vi "Main.vi"(11 "Module Admin":refnum<class "Delacor_lib_QMH_Module Admin.lvclass">) -> ()   [LabVIEW 2023, in "horiba.lvlib" / "LiveLogger.lvlib"]
doc: "This template is based off of the Queued Message Handler design pattern and the Queued Message Handler project template that ships with LabVIEW.\n\nThe main difference is that the queue is private to this module and communication between modules is performed via Broadcast and Request events.\n\nRequest events are wrapped in public API methods and are handled in the Event Handling Loop (EHL) of this VI. Any module can register for Broadcast events sent by this module. The EHL generates messages based on user interface actions.\n\nThe Message Handling Loop (MHL) processes messages generated by the EHL, or by other messages. The messages are string values, so new messages can be added easily to the Message Cases case structure in the MHL. Each message cluster can also provide an optional value for Message Data, which is a variant that can be converted to whatever message-specific data is required.\n_____\nBased on DQMH Project Template 7.0.1.1316."
uses:
  LiveLogger.lvlib
  <vilib>/Delacor/Delacor QMH/Libraries/Module Admin_class/Delacor_lib_QMH_Module Admin.lvclass
  <vilib>/QSI/QControls/QControl Classes/RichTextBox/Bold Button.ctl
  <vilib>/QSI/QControls/QControl Classes/RichTextBox/Italic Button.ctl
  <vilib>/QSI/QControls/QControl Classes/RichTextBox/Underline Button.ctl
  <vilib>/QSI/QControls/QControl Classes/RichTextBox/Strikethrough Button.ctl
  <vilib>/QSI/QControls/QControl Classes/RichTextBox/Justification.ctl
  <vilib>/QSI/QControls/QControl Classes/RichTextBox/Align Left Button.ctl
  <vilib>/QSI/QControls/QControl Classes/RichTextBox/Align Center Button.ctl
  <vilib>/QSI/QControls/QControl Classes/RichTextBox/Align Right Button.ctl
  <vilib>/QSI/QControls/QControl Classes/RichTextBox/Toggle Codes Button.ctl
  <vilib>/Hampel Software Engineering/HSE Logger/LogLevel.ctl
  Module Data--cluster.ctl
  <vilib>/Delacor/Delacor QMH/Libraries/Message Queue_class/Delacor_lib_QMH_Message Queue.lvclass/Delacor_lib_QMH_Message Queue.ctl
  Stop Argument--cluster.ctl
  <vilib>/Delacor/Delacor QMH/Libraries/Module Admin_class/Delacor_lib_QMH_Module Admin.lvclass/Delacor_lib_QMH_Module Admin.ctl
  <vilib>/Utility/miscctls.llb/LVPointTypeDef.ctl
  <vilib>/Delacor/Delacor QMH/Libraries/Message Queue_class/Delacor_lib_QMH_Enqueue Message (Single).vi
  <vilib>/Delacor/Delacor QMH/Libraries/Module Admin_class/Delacor_lib_QMH_Get External Launch.vi
  <vilib>/Hampel Software Engineering/HSE Logger/Handler/UserEventHandler/UserEventHandler.lvclass
  <vilib>/QSI/QControls/QControl Classes/RichTextBox/RichTextBox.lvclass
  <vilib>/QSI/QControls/QControl Classes/RichTextBox/Write Tagged String.vi
  <vilib>/Delacor/Delacor QMH/Libraries/Message Queue_class/Delacor_lib_QMH_Message Queue.lvclass
  <vilib>/Hampel Software Engineering/HSE Logger/hse-logger.lvlib
panel:
  in  "Autoscroll?":bool
  in  "Toolbar":T7
  in  "RichTextBox":string
  in  "Stop":bool
  out "error out":errorcluster
  in  "Simulate MHL Error":bool
  in  "Simulate EHL Error":bool
  # "Connector Pane"
  # "Locals"
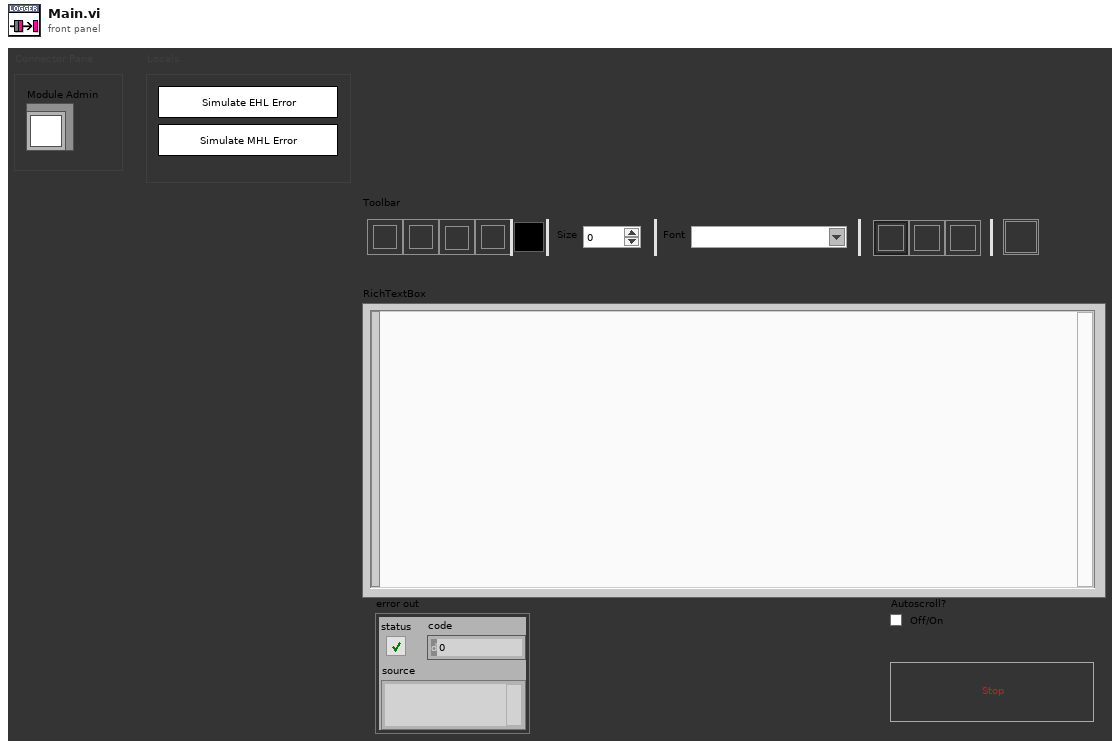
[diagram p1: front panel]
types:
  T1 = typedef "RichTextBox.lvclass/Bold Button.ctl" = bool
  T2 = typedef "RichTextBox.lvclass/Italic Button.ctl" = bool
  T3 = typedef "RichTextBox.lvclass/Underline Button.ctl" = bool
  T4 = typedef "RichTextBox.lvclass/Strikethrough Button.ctl" = bool
  T5 = typedef "RichTextBox.lvclass/Justification.ctl" = enum32{"Left", "Center", "Right"}
  T6 = typedef "RichTextBox.lvclass/Toggle Codes Button.ctl" = bool
  T7 = cluster{"Bold Button":T1, "Italic Button":T2, "Underline Button":T3, "Strikeout Button":T4, "Text Color":u32, "Size":u32, "Font":string, "Justification":T5, "Toggle Codes":T6}
  T8 = typedef "hse-logger.lvlib/LogLevel.ctl" = enum16{"DEBUG", "INFO", "WARNING", "ERROR", "CRITICAL"}
  T9 = typedef "horiba.lvlib/LiveLogger.lvlib/Request Events--cluster.ctl" = cluster{"Stop Module":refnum<user-event>, "Show Panel":refnum<user-event>, "Hide Panel":refnum<user-event>, "Get Module Execution Status":refnum<user-event>, "Show Diagram":refnum<user-event>}
  T10 = typedef "horiba.lvlib/LiveLogger.lvlib/Module Data--cluster.ctl" = cluster{"Status":string}
  T11 = enum32{"invalid lock state", "Not Locked", "Locked (No Password)", "Password-protected"}
  T12 = typedef "horiba.lvlib/LiveLogger.lvlib/Stop Argument--cluster.ctl" = cluster{"Origin":string, "Exit via Stop Module Req?":bool, "Wait for Module to stop?":bool}
  T13 = typedef "LVPointTypeDef.ctl" = cluster{"Horizontal":i16, "Vertical":i16}
  T14 = enum32{"Invalid", "Standard", "Closed", "Hidden", "Minimized", "Maximized"}
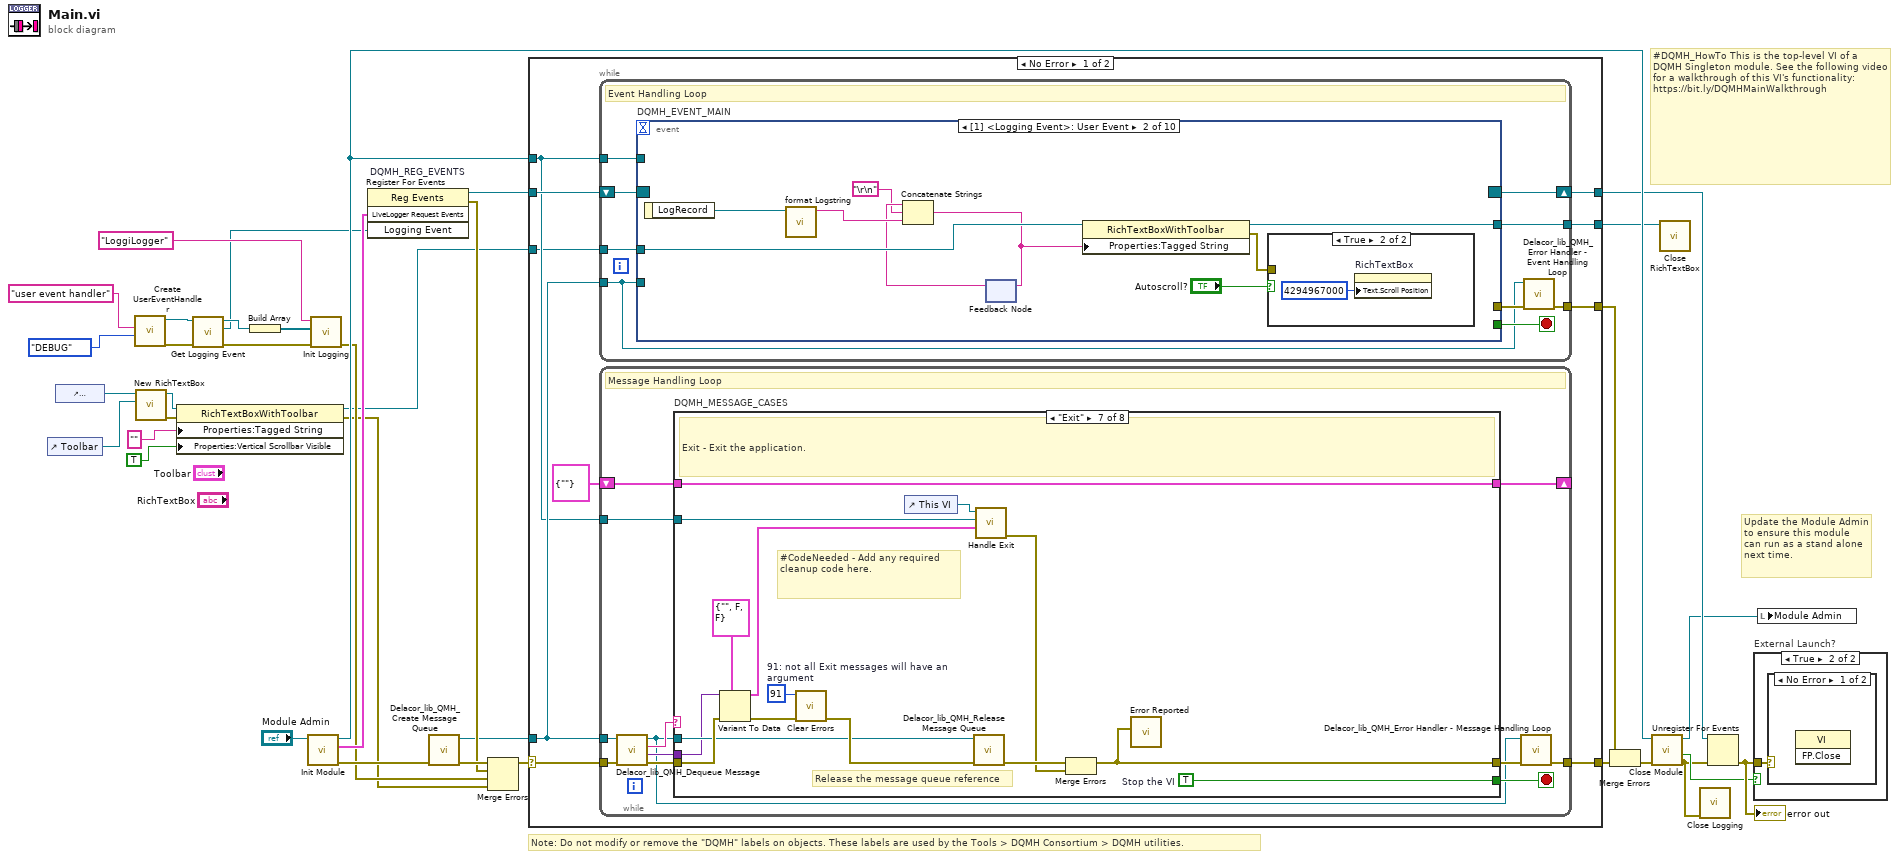
[diagram p0: block diagram]
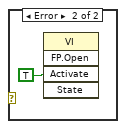
[diagram p3: hidden frame]
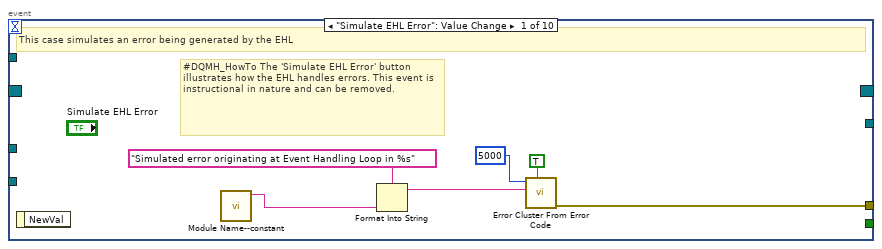
[diagram p4: hidden frame]
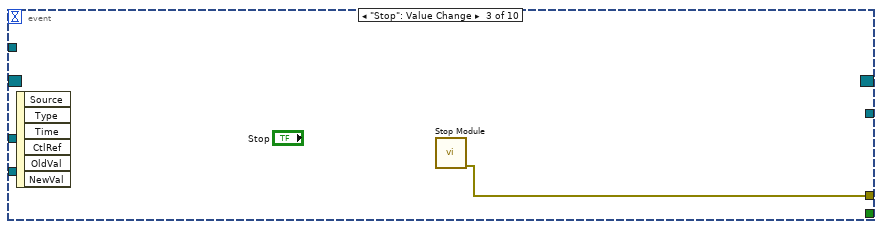
[diagram p6: hidden frame]
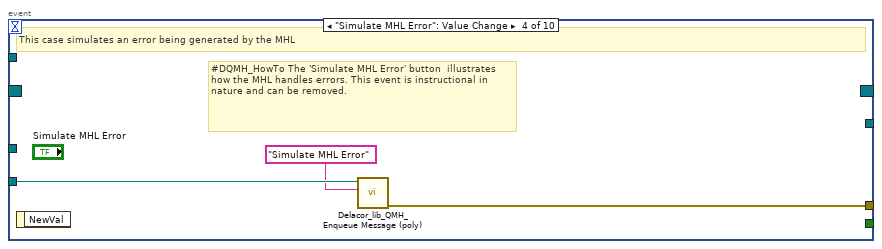
[diagram p7: hidden frame]
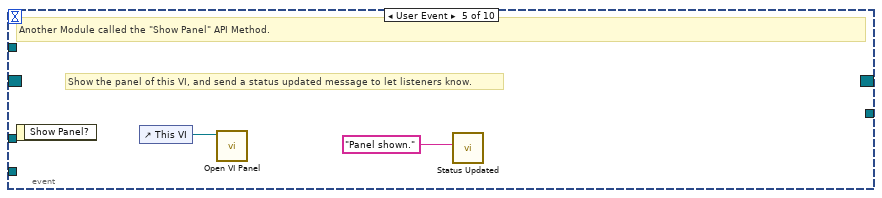
[diagram p8: hidden frame]
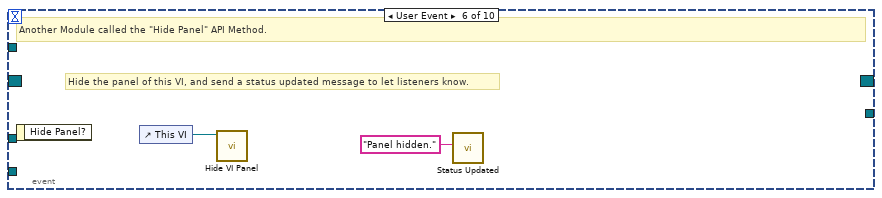
[diagram p9: hidden frame]
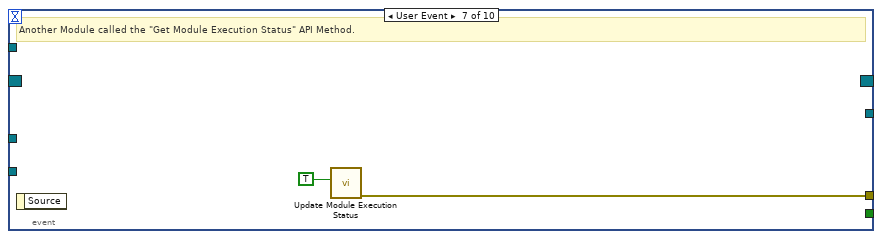
[diagram p10: hidden frame]
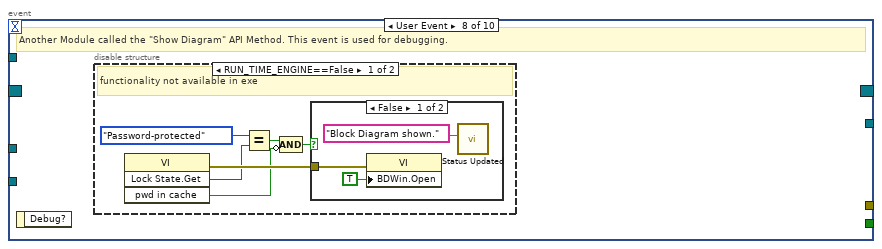
[diagram p11: hidden frame]
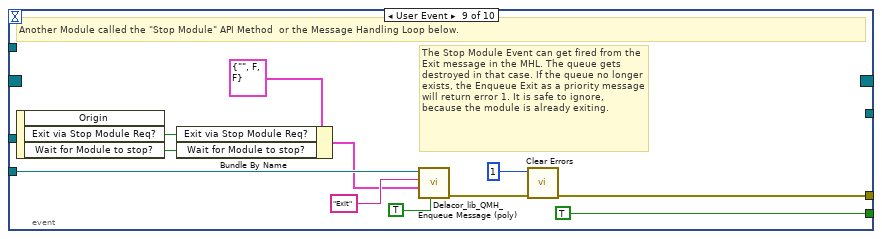
[diagram p14: hidden frame]
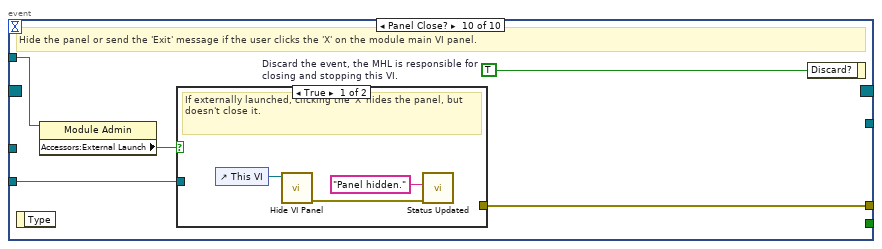
[diagram p15: hidden frame]
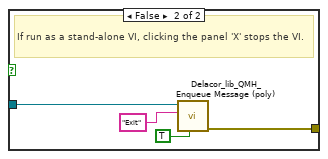
[diagram p16: hidden frame]
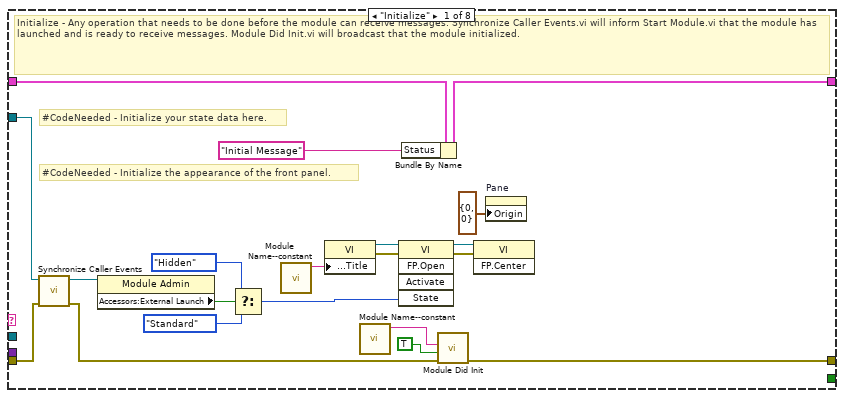
[diagram p17: hidden frame]
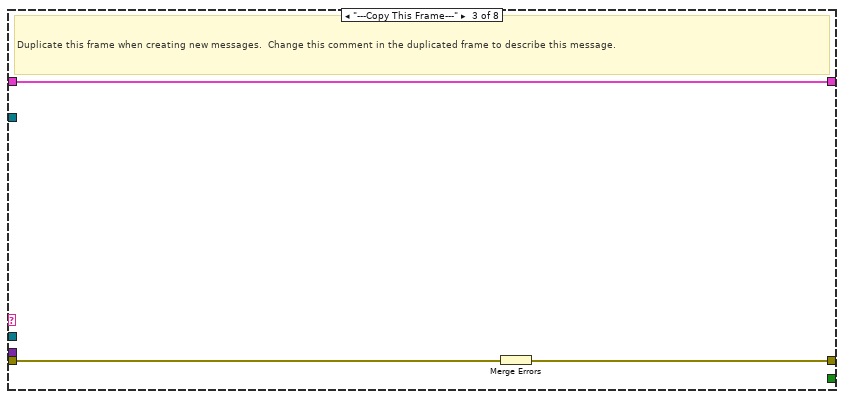
[diagram p19: hidden frame]
diagram:
  # "#DQMH_HowTo This is the top-level VI of a DQMH Singleton module. See the following video for a walkthrough of this VI's functionality: https://bit.ly/DQMHMainWalkthrough"
  # "Note: Do not modify or remove the \"DQMH\" labels on objects. These labels are used by the Tools > DQMH Consortium > DQMH utilities."
  # "Update the Module Admin to ensure this module can run as a stand alone next time."
  n1 = control-ref of="Toolbar"() -> (w8:refnum<vi>)
  n2 = control-ref of="RichTextBox"() -> (w9:refnum<vi>)
  n3 = call <vilib>:"Create UserEventHandler.vi"("Level"=LogLevel."DEBUG", "Name"="user event handler") -> ("error out"=w15:errorcluster, "UserEventHandler out"=w16:refnum<class "UserEventHandler.lvclass">)  [unwired: 8 in]
  n4 = call <vilib>:"New RichTextBox.vi"("ToolbarReference"=w8, "Reference"=w9) -> ("error out"=w7:errorcluster, "RichTextBox out"=w6:refnum<class "RichTextBox.lvclass">)  [unwired: 7 in, 1 out]
  n5 = property class="RichTextBoxWithToolbar"(reference=w6, error in=w7, "Properties:Tagged String"="" ("Status"), "Properties:Vertical Scrollbar Visible"=TRUE ("Vertical Scrollbar Visible")) -> (reference out=w3:refnum<class "RichTextBox.lvclass">, error out=w5:errorcluster)
  n6 = call-dynamic "Get Logging Event.vi"("error in"=w15, "UserEventHandler in"=w16) -> ("error out"=w14:errorcluster, "Logging Event"=w12:refnum<user-event>, "UserEventHandler out"=w13:refnum<class "UserEventHandler.lvclass">)  [unwired: 7 in]
  n7 = Build Array(w13) -> (w19:refnum<class "UserEventHandler.lvclass">[])
  n8 = call "Init Module.vi"("Singleton Module Admin in"="Module Admin") -> ("error out"=w35:errorcluster, "LiveLogger Request Events"=w25:T9, "Singleton Module Admin out"=w28:refnum<class "Delacor_lib_QMH_Module Admin.lvclass">)  [unwired: 8 in]
  n9 = call <vilib>:"Init Logging.vi"("error in"=w14, "Handlers"=w19, "Name"="LoggiLogger") -> ("error out"=w11:errorcluster)  [unwired: 8 in]
  n10 = register-events "DQMH_REG_EVENTS"(w25, w12) -> (reference out=w26:refnum<event-registration>, error out=w29:errorcluster)  [unwired: 2 in]
  n11 = call <vilib>:"Delacor_lib_QMH_Create Message Queue.vi"("error in"=w35) -> ("error out"=w31:errorcluster, "Message Queue"=w24:refnum<class "Delacor_lib_QMH_Message Queue.lvclass">)  [unwired: 9 in]
  n12 = Merge Errors(w31, w29, w11, w5) -> (w30:errorcluster)
  n13 = case shown="No Error" w30 {
    selector: w30 -> [w44 w212]
    tunnel: [w46 w211] -> w36
    tunnel: [w43 w210] -> w27
    tunnel: w26 -> [w41 w210]
    tunnel: w24 -> [w40 w205]
    tunnel: [w45 _] -> w34
    tunnel: w28 -> [w39 w206]
    tunnel: w3 -> [w38 w204]
    tunnel: [w37 w204] -> w2
    frame No Error {
      n14 = while {
        tunnel: w40 -> [w49]
        shift-right: [w52] -> w43
        shift-left: w41 -> [w53]
        tunnel: [w54] -> w45
        tunnel: w39 -> [w50]
        tunnel: w38 -> [w48]
        tunnel: [w47] -> w37
        stop <- w51 stop-if-true
        # "Event Handling Loop"
        n15 = event "DQMH_EVENT_MAIN" shown="[1] <Logging Event>: User Event" {
          selector: w53 -> [_ _ _ _ _ _ _ _ _ _]
          dyn-events: [_ _ _ _ _ _ _ _ _ _] -> w52
          timeout: _ -> [_ _ _ _ _ _ _ _ _ _]
          tunnel: [_ _ _ _ _ _ _ _ TRUE ("Discard?") _] -> w51
          tunnel: w49 -> [_ _ _ w74 _ _ _ _ w97 w104]
          tunnel: [w61 _ w72 w75 _ _ w81 _ w100 w106] -> w55
          tunnel: w50 -> [_ _ _ _ _ _ _ _ _ w103]
          tunnel: w48 -> [_ w68 _ _ _ _ _ _ _ _]
          tunnel: [_ w64 _ _ _ _ _ _ _ _] -> w47
          event "Simulate EHL Error": Value Change {
            # "#DQMH_HowTo The 'Simulate EHL Error' button  illustrates how the EHL handles errors. This event is instructional in nature and can be removed."
            # "This case simulates an error being generated by the EHL"
            n16 = event-data() -> ()  [unwired: 1 in, 1 out]
            n17 = call "Module Name--constant.vi"() -> ("Module Name"=w58:string)  [unwired: 11 in]
            n18 = Format Into String(format string="Simulated error originating at Event Handling Loop in %s", w58) -> (resulting string=w59:string)  [unwired: 2 in, 1 out]
            n19 = call <vilib>:"Error Cluster From Error Code.vi"("show call chain? (False)"=TRUE, "error message (\"\")"=w59, "error code (0)"=5000) -> ("error out"=w61:errorcluster)  [unwired: 6 in]
          }
          event User Event {
            n20 = event-data() -> ("LogRecord"=w70:refnum<class "LogRecord.lvclass">)  [unwired: 1 in]
            n21 = call "format Logstring.vi"("LogRecord in"=w70) -> ("LogLine"=w69:string)  [unwired: 10 in]
            n22 = feedback #1() -> (w67:string)  [unwired: 1 in]
            n23 = Concatenate Strings(w67, "\r\n", w69) -> (w65:string)
            n24 = feedback-in #1(w65) -> ()
            n25 = property class="RichTextBoxWithToolbar"(reference=w68, "Properties:Tagged String"=w65) -> (reference out=w64:refnum<class "RichTextBox.lvclass">, error out=w62:errorcluster)  [unwired: 1 in]
            n26 = case shown="True" "Autoscroll?" {
              tunnel: w62 -> [_ _]
              frame False {
              }
              frame True {
                n27 = property on="RichTextBox" class="Str"("Text.Scroll Position"=u32 4294967000) -> ()  [unwired: 2 in, 2 out]
              }
            }
          }
          event "Stop": Value Change {
            n28 = event-data() -> ()  [unwired: 1 in, 6 out]
            n29 = call "Stop Module.vi"() -> ("error out"=w72:errorcluster)  [unwired: 11 in]
          }
          event "Simulate MHL Error": Value Change {
            # "#DQMH_HowTo The 'Simulate MHL Error' button  illustrates how the MHL handles errors. This event is instructional in nature and can be removed."
            # "This case simulates an error being generated by the MHL"
            n30 = event-data() -> ()  [unwired: 1 in, 1 out]
            n31 = call-poly <vilib>:"Delacor_lib_QMH_Enqueue Message (poly).vi"("Message"="Simulate MHL Error", "Message Queue in"=w74) -> ("error out"=w75:errorcluster)  [unwired: 8 in, 1 out]
          }
          event User Event {
            # "Show the panel of this VI, and send a status updated message to let listeners know."
            # "Another Module called the \"Show Panel\" API Method."
            n32 = event-data() -> ()  [unwired: 1 in, 1 out]
            n33 = control-ref of="This VI"() -> (w77:refnum<vi>)
            n34 = call "Open VI Panel.vi"("VI"=w77) -> ()  [unwired: 10 in, 1 out]
            n35 = call "Status Updated.vi"("Status"="Panel shown." ("format string")) -> ()  [unwired: 10 in, 1 out]
          }
          event User Event {
            # "Hide the panel of this VI, and send a status updated message to let listeners know."
            # "Another Module called the \"Hide Panel\" API Method."
            n36 = event-data() -> ()  [unwired: 1 in, 1 out]
            n37 = control-ref of="This VI"() -> (w79:refnum<vi>)
            n38 = call "Hide VI Panel.vi"("VI"=w79) -> ()  [unwired: 10 in, 1 out]
            n39 = call "Status Updated.vi"("Status"="Panel hidden." ("format string")) -> ()  [unwired: 10 in, 1 out]
          }
          event User Event {
            # "Another Module called the \"Get Module Execution Status\" API Method."
            n40 = event-data() -> ()  [unwired: 1 in, 1 out]
            n41 = call "Update Module Execution Status.vi"("Running?"=TRUE) -> ("error out"=w81:errorcluster)  [unwired: 10 in]
          }
          event User Event {
            # "Another Module called the \"Show Diagram\" API Method. This event is used for debugging."
            n42 = event-data() -> ()  [unwired: 1 in, 1 out]
            n43 = disable-structure shown="RUN_TIME_ENGINE==False" {
              frame condition #0 (active) {
                # "functionality not available in exe"
                n44 = invoke on="Invoke Node" class="VI" method="Lock State.Get"() -> (error out=w87:errorcluster, "Get Lock State"=w86:T11, "pwd in cache"=w83:bool)  [unwired: 4 in, 1 out]
                n45 = Equal?(x=T11."Password-protected", y=w86) -> (x = y?=w84:bool)
                n46 = Compound Arithmetic op=AND(w84, invert w83) -> (w82:bool)
                n47 = case shown="False" w82 {
                  tunnel: w87 -> [w90 _]
                  frame False {
                    n48 = property on="Property Node" class="VI"(error in=w90, "BDWin.Open"=TRUE ("Block Diagram Window:Open")) -> ()  [unwired: 1 in, 2 out]
                    n49 = call "Status Updated.vi"("Status"="Block Diagram shown." ("format string")) -> ()  [unwired: 10 in, 1 out]
                  }
                  frame True {
                    # "Password-protected VI, and the password is not in the cache. Do not show the diagram."
                  }
                }
              }
              frame condition #1 {
              }
            }
          }
          event User Event {
            # "The Stop Module Event can get fired from the Exit message in the MHL. The queue gets destroyed in that case. If the queue no longer exists, the Enqueue Exit as a priority message will return error 1. It is safe to ignore, because the module is already exiting."
            # "Another Module called the \"Stop Module\" API Method  or the Message Handling Loop below."
            n50 = event-data() -> ("Exit via Stop Module Req?"=w93:bool, "Wait for Module to stop?"=w92:bool)  [unwired: 1 in, 1 out]
            n51 = Bundle By Name(cluster=T12 {"Origin"="", "Exit via Stop Module Req?"=FALSE, "Wait for Module to stop?"=FALSE} ("Stop Argument"), "Exit via Stop Module Req?"=w93, "Wait for Module to stop?"=w92) -> (w91:T12)
            n52 = call-poly <vilib>:"Delacor_lib_QMH_Enqueue Message (poly).vi"("Priority Message? (F)"=TRUE, "Message Data"=w91, "Message"="Exit", "Message Queue in"=w97) -> ("error out"=w101:errorcluster)  [unwired: 6 in, 1 out]
            n53 = call <vilib>:"Clear Errors.vi"("error in (no error)"=w101, "specific error code to clear (0: all)"=1) -> ("error out"=w100:errorcluster)  [unwired: 4 in, 1 out]
          }
          event Panel Close? {
            w105 = TRUE  # Discard the event, the MHL is responsible for closing and stopping this VI.
            # "Hide the panel or send the 'Exit' message if the user clicks the 'X' on the module main VI panel."
            n54 = event-data() -> ()  [unwired: 1 in, 1 out]
            n55 = property on="Property Node" class="Module Admin"(reference=w103) -> ("Accessors:External Launch"=w102:bool)  [unwired: 1 in, 2 out]
            n56 = case shown="True" w102 {
              tunnel: w104 -> [_ w112]
              tunnel: [_ w113] -> w106
              frame True {
                # "If externally launched, clicking the 'X' hides the panel, but doesn't close it."
                n57 = control-ref of="This VI"() -> (w109:refnum<vi>)
                n58 = call "Hide VI Panel.vi"("VI"=w109) -> ("error out"=w107:errorcluster)  [unwired: 10 in]
                n59 = call "Status Updated.vi"("error in"=w107, "Status"="Panel hidden." ("format string")) -> ()  [unwired: 9 in, 1 out]
              }
              frame False {
                # "If run as a stand-alone VI, clicking the panel 'X' stops the VI."
                n60 = call-poly <vilib>:"Delacor_lib_QMH_Enqueue Message (poly).vi"("Priority Message? (F)"=TRUE, "Message"="Exit", "Message Queue in"=w112) -> ("error out"=w113:errorcluster)  [unwired: 7 in, 1 out]
              }
            }
            n61 = event-data ("Event Filter Node")("Discard?"=w105) -> ()  [unwired: 1 in, 1 out]
          }
        }
        n62 = call-dynamic "Delacor_lib_QMH_Error Handler - Event Handling Loop.vi"("error in"=w55, "Message Queue in"=w49) -> ("dup error in"=w54:errorcluster)  [unwired: 8 in, 1 out]
      }
      n63 = while {
        tunnel: w40 -> [w114]
        shift-right: [w122] -> _
        shift-left: T10 {"Status"=""} ("Data Cluster") -> [w123]
        tunnel: w44 -> [w125]
        tunnel: [w117] -> w46
        tunnel: w39 -> [w118]
        stop <- w121 stop-if-true
        # "Message Handling Loop"
        n64 = call-dynamic "Delacor_lib_QMH_Dequeue Message.vi"("error in"=w125, "Message Queue in"=w114) -> ("error out"=w124:errorcluster, "Message Data"=w119:variant, "Message"=w120:string, "Message Queue out"=w115:refnum<class "Delacor_lib_QMH_Message Queue.lvclass">)  [unwired: 6 in]
        n65 = case "DQMH_MESSAGE_CASES" shown="\"Exit\"" w120 {
          selector: w120 -> [_ _ _ _ _ _ _ w199]
          tunnel: w115 -> [_ _ _ _ _ w165 w187 _]
          tunnel: w124 -> [w143 w147 w150 w152 w161 w172 w193 w202]
          tunnel: [w141 w147 w149 w152 w160 w168 w188 w203] -> w116
          tunnel: w123 -> [w132 w146 w148 w151 w158 w167 w186 w200]
          tunnel: [w131 w146 w148 w151 w158 w167 w186 w200] -> w122
          tunnel: [_ _ _ _ _ _ w185 _] -> w121
          tunnel: w119 -> [_ _ _ _ _ w166 w184 _]
          tunnel: w118 -> [w133 _ _ _ _ w164 w179 _]
          frame "Initialize" {
            # "#CodeNeeded - Initialize the appearance of the front panel."
            # "#CodeNeeded - Initialize your state data here."
            # "Initialize - Any operation that needs to be done before the module can receive messages. Synchronize Caller Events.vi will inform Start Module.vi that the module has launched and is ready to receive messages. Module Did Init.vi will broadcast that the module initialized."
            n66 = call "Synchronize Caller Events.vi"("error in"=w143, "Singleton Module Admin in"=w133) -> ("error out"=w142:errorcluster, "Singleton Module Admin out"=w128:refnum<class "Delacor_lib_QMH_Module Admin.lvclass">)  [unwired: 8 in]
            n67 = property on="Property Node" class="Module Admin"(reference=w128) -> ("Accessors:External Launch"=w137:bool)  [unwired: 1 in, 2 out]
            n68 = Select(t=T14."Hidden" ("State"), s=w137, f=T14."Standard" ("State")) -> (s? t:f=w134:T14)
            n69 = call "Module Name--constant.vi"() -> ("Module Name"=w140:string)  [unwired: 11 in]
            n70 = property on="Property Node" class="VI"("Front Panel.Title"=w140) -> (reference out=w139:refnum<vi>, error out=w145:errorcluster)  [unwired: 2 in]
            n71 = call "Module Name--constant.vi"() -> ("Module Name"=w129:string)  [unwired: 11 in]
            n72 = invoke on="Invoke Node" class="VI" method="FP.Open"(reference=w139, error in=w145, "State"=w134) -> (reference out=w138:refnum<vi>, error out=w144:errorcluster)  [unwired: 2 in, 3 out]
            n73 = Bundle By Name(cluster=w132, "Status"="Initial Message" ("Initial Message")) -> (w131:T10)
            n74 = call "Module Did Init.vi"("error in"=w142, "Initialized?"=TRUE, "Origin"=w129) -> ("error out"=w141:errorcluster)  [unwired: 8 in]
            n75 = invoke on="Invoke Node" class="VI" method="FP.Center"(reference=w138, error in=w144) -> ()  [unwired: 1 in, 3 out]
            n76 = property on="Pane" class="Pane"("Origin"=T13 {"Horizontal"=0, "Vertical"=0}) -> ()  [unwired: 2 in, 2 out]
          }
          frame "---Module Specific---" {
            # "Separator -- The following cases handle messages specific to this Module."
          }
          frame "---Copy This Frame---" {
            # "Duplicate this frame when creating new messages.  Change this comment in the duplicated frame to describe this message."
            n77 = Merge Errors(w150) -> (w149:errorcluster)
          }
          frame "---Exit and Error Handling---" {
            # "Separator - The following cases handle errors and exit messages."
          }
          frame "Simulate MHL Error" {
            # "#DQMH_HowTo The 'Simulate MHL Error' button  illustrates how the MHL handles errors. This event is instructional in nature and can be removed."
            # "Simulate an error occurring at the MHL"
            n78 = call "Module Name--constant.vi"() -> ("Module Name"=w154:string)  [unwired: 11 in]
            n79 = Format Into String(format string="Simulated error originating at Message Handling Loop in %s", w154) -> (resulting string=w155:string)  [unwired: 2 in, 1 out]
            n80 = call <vilib>:"Error Cluster From Error Code.vi"("show call chain? (False)"=TRUE, "error message (\"\")"=w155, "error code (0)"=5001) -> ("error out"=w159:errorcluster)  [unwired: 6 in]
            n81 = Merge Errors(w161, w159) -> (w160:errorcluster)
          }
          frame "Error" {
            # "#CodeRecommended - If the module is running in standalone mode (External Launch = FALSE), this code will pop up an error dialog and call the 'Exit' message if an error occurs. Add more fine-grained error management here."
            # "Error - Check the error message data and respond accordingly. This message is sent by the \"Error Handler\" VIs at the end of each loop in this application."
            n82 = property on="Property Node" class="Module Admin"(reference=w164) -> ("Accessors:External Launch"=w163:bool)  [unwired: 1 in, 2 out]
            n83 = Variant To Data(error in=w172, type=errorcluster {"status"=FALSE, "code"=0, "source"=""} ("error constant"), Variant=w166) -> (data=w162:errorcluster, error out=w170:errorcluster)
            n84 = local write "error out"(w162) -> ()
            n85 = call "Error Reported.vi"("Error"=w162) -> ()  [unwired: 10 in, 1 out]
            n86 = case shown="False" w163 {
              tunnel: [w177 _] -> w169
              tunnel: w165 -> [w175 _]
              tunnel: w162 -> [w176 _]
              frame False {
                n87 = disable-structure shown="Default" {
                  disable-tunnel: w176 -> [w178 _]
                  frame condition #0 (active) {
                    # "If the module is running standalone, then pop up an error dialog and call the \"Exit\" message."
                    n88 = call <vilib>:"Simple Error Handler.vi"("error in (no error)"=w178) -> ()  [unwired: 4 in, 5 out]
                  }
                  frame condition #1 {
                    # "To prevent the Simple Error Handler VI from being loaded (e.g. when deploying to a Real-Time target), add the Conditional Disable Symbol \"DQMH_Disable_SEH\" to your project and set it to TRUE."
                  }
                }
                n89 = call-poly <vilib>:"Delacor_lib_QMH_Enqueue Message (poly).vi"("Priority Message? (F)"=TRUE, "Message"="Exit", "Message Queue in"=w175) -> ("error out"=w177:errorcluster)  [unwired: 7 in, 1 out]
              }
              frame True {
                # "If the module was launched externally, calling the Error Reported broadcast VI is the only action performed by the \"Error\" message. The module's caller can then process the error appropriately."
              }
            }
            n90 = Merge Errors(w170, w169) -> (w168:errorcluster)
          }
          frame "Exit" {
            w183 = 91  # 91: not all Exit messages will have an argument
            w185 = TRUE  # Stop the VI
            # "Release the message queue reference"
            # "#CodeNeeded - Add any required cleanup code here."
            # "Exit - Exit the application."
            n91 = Variant To Data(error in=w193, type=T12 {"Origin"="", "Exit via Stop Module Req?"=FALSE, "Wait for Module to stop?"=FALSE} ("Stop Argument"), Variant=w184) -> (data=w181:T12, error out=w190:errorcluster)
            n92 = call <vilib>:"Clear Errors.vi"("error in (no error)"=w190, "specific error code to clear (0: all)"=w183) -> ("error out"=w192:errorcluster)  [unwired: 4 in, 1 out]
            n93 = control-ref of="This VI"() -> (w180:refnum<vi>)
            n94 = call-dynamic "Delacor_lib_QMH_Release Message Queue.vi"("error in"=w192, "Message Queue"=w187) -> ("error out"=w191:errorcluster)  [unwired: 9 in]
            n95 = call "Handle Exit.vi"("Stop Argument"=w181, "Admin in"=w179, "VI reference"=w180) -> ("error out"=w189:errorcluster)  [unwired: 7 in, 1 out]
            n96 = Merge Errors(w191, w189) -> (w188:errorcluster)
            n97 = call "Error Reported.vi"("Error"=w188) -> ()  [unwired: 10 in, 1 out]
          }
          frame Default {
            # "'Default' case only runs if there is a message that isn't defined in any of the other cases.  Output a programming error."
            n98 = call "Module Name--constant.vi"() -> ("Module Name"=w198:string)  [unwired: 11 in]
            n99 = Format Into String(format string="The invalid message string \"%s\" was received in the Message Handling Loop for module \"%s\".", w199, w198) -> (resulting string=w194:string)  [unwired: 2 in, 1 out]
            n100 = call <vilib>:"Error Cluster From Error Code.vi"("show call chain? (False)"=TRUE, "error message (\"\")"=w194, "error code (0)"=1) -> ("error out"=w201:errorcluster)  [unwired: 6 in]
            n101 = Merge Errors(w202, w201) -> (w203:errorcluster)
          }
        }
        n102 = call-dynamic "Delacor_lib_QMH_Error Handler - Message Handling Loop.vi"("error in"=w116, "Message Queue in"=w115) -> ("dup error in"=w117:errorcluster)  [unwired: 8 in, 1 out]
      }
    }
    frame Error {
      # "Synchronize Caller Events.vi will inform Start Module.vi that the module has launched and will let the code calling Start Module.vi register for broadcasts and would permit the caller receive the broadcast that an error occurred at launch time."
      n103 = call-dynamic "Delacor_lib_QMH_Release Message Queue.vi"("error in"=w212, "Message Queue"=w205) -> ("error out"=w211:errorcluster)  [unwired: 9 in]
      n104 = call "Synchronize Caller Events.vi"("Singleton Module Admin in"=w206) -> ("error out"=w213:errorcluster)  [unwired: 9 in, 1 out]
      n105 = call "Module Name--constant.vi"() -> ("Module Name"=w209:string)  [unwired: 11 in]
      n106 = Format Into String(format string="An error occurred during initialization. %s is no longer running.", w209) -> (resulting string=w207:string)  [unwired: 2 in, 1 out]
      n107 = Merge Errors(w211, w213) -> (w214:errorcluster)
      n108 = call "Error Reported.vi"("Additional Information"=w207, "Error"=w214) -> ()  [unwired: 9 in, 1 out]
    }
  }
  n109 = Merge Errors(w34, w36) -> (w33:errorcluster)
  n110 = call "Close Module.vi"("error in"=w33, "Module Admin in"=w28) -> ("error out"=w10:errorcluster, "External Launch"=w21:bool, "Module Admin out"=w22:refnum<class "Delacor_lib_QMH_Module Admin.lvclass">)  [unwired: 7 in]
  n111 = call <vilib>:"Close RichTextBox.vi"("RichTextBox in"=w2) -> ()  [unwired: 10 in, 1 out]
  n112 = call <vilib>:"Close Logging.vi"("error in"=w10) -> ()  [unwired: 10 in, 1 out]
  n113 = Unregister For Events(event registration refnum=w27, error in=w10) -> (error out=w32:errorcluster)
  "error out" <- w32
  n114 = case "External Launch?" shown="True" w21 {
    tunnel: w32 -> [_ w215]
    frame False {
    }
    frame True {
      n115 = case shown="No Error" w215 {
        frame No Error {
          n116 = invoke on="Invoke Node" class="VI" method="FP.Close"() -> ()  [unwired: 3 in, 3 out]
        }
        frame Error {
          n117 = invoke on="Invoke Node" class="VI" method="FP.Open"("Activate"=TRUE ("Activate?")) -> ()  [unwired: 4 in, 5 out]
        }
      }
    }
  }
  n118 = local write "Module Admin"(w22) -> ()
